vi "Rename VI.vi"(6 "Rename":string, 8 "error in":errorcluster, 9 "VI Name":string, 10 "Owned Items[]":refnum<vi>[](array[refnum])) -> (0 "error out":errorcluster)   [LabVIEW 2025, in "_Rename.lvlib" / "_Rename.lvclass"]
uses:
  _Rename.lvclass
  _Rename.lvclass/_Rename.ctl
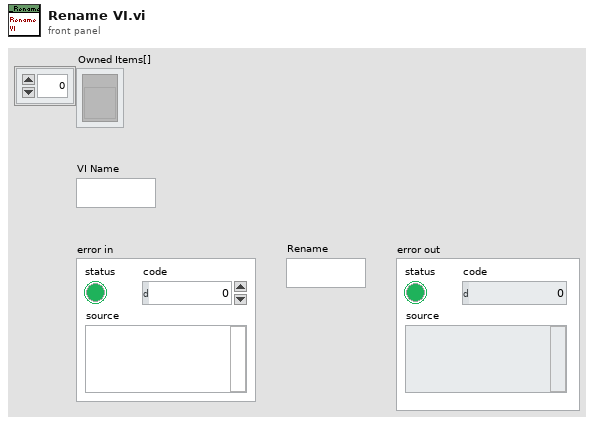
[diagram p1: front panel]
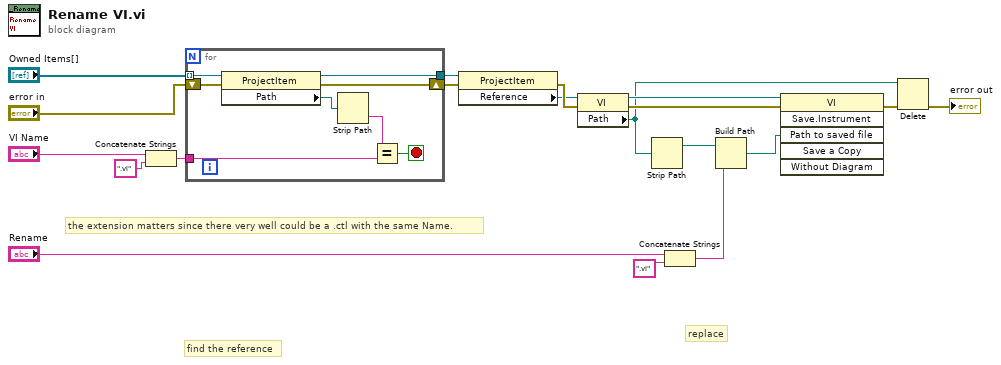
[diagram p0: block diagram]
diagram:
  # "replace"
  # "find the reference"
  # "the extension matters since there very well could be a .ctl with the same Name."
  # "the extension matters since there very well could be a .ctl with the same Name."
  n1 = Concatenate Strings("VI Name", ".vi" ("string")) -> (w17:string)
  n2 = for {
    tunnel: "Owned Items[]" -> [w27] mode=indexing
    shift-right: [w25] -> w18
    shift-left: "error in" -> [w26]
    tunnel: [w24] -> w19
    tunnel: w17 -> [w20]
    stop <- w23 stop-if-true
    n3 = property class="ProjectItem"(reference=w27, error in=w26) -> (reference out=w24:refnum<vi>, error out=w25:errorcluster, "Path"=w22:path)
    n4 = Strip Path(path=w22) -> (name=w21:string)  [unwired: 1 out]
    n5 = Equal?(x=w21, y=w20) -> (x = y?=w23:bool)
  }
  n6 = property class="ProjectItem"(reference=w19, error in=w18) -> (error out=w4:errorcluster, "Reference"=w3:refnum<vi>)  [unwired: 1 out]
  n7 = property class="VI"(reference=w3, error in=w4) -> (reference out=w7:refnum<vi>, error out=w8:errorcluster, "Path"=w6:path)
  n8 = Strip Path(path=w6) -> (stripped path=w11:path)  [unwired: 1 out]
  n9 = Concatenate Strings("Rename", ".vi" ("string")) -> (w9:string)
  n10 = Build Path(base path=w11, name or relative path=w9) -> (appended path=w12:path)
  n11 = invoke class="VI" method="Save.Instrument"(reference=w7, error in=w8, "Path to saved file"=w12) -> (error out=w5:errorcluster)  [unwired: 3 in, 5 out]
  n12 = Delete(path (use dialog)=w6, error in=w5) -> (error out=→"error out":errorcluster)  [unwired: 3 in, 2 out]
